vi "move.vi"(8 "error in (no error)":errorcluster, 11 "StageMG100204SutterMP285 in":refnum<class "StageMG100204SutterMP285.lvclass">=refnum) -> (0 "error out":errorcluster, 3 "StageMG100204SutterMP285 out":refnum<class "StageMG100204SutterMP285.lvclass">)   [LabVIEW 2010, in "StageMG100204SutterMP285.lvclass"]
uses:
  StageMG100204SutterMP285.lvclass
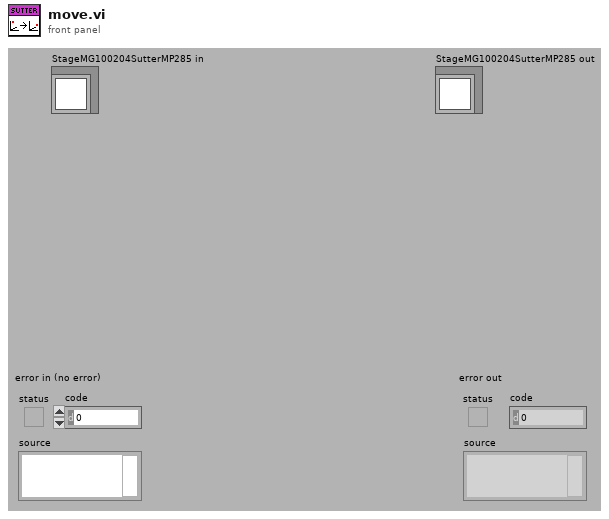
[diagram p1: front panel]
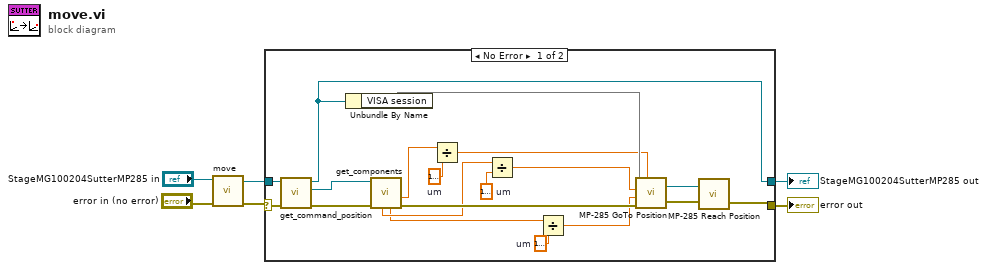
[diagram p0: block diagram]
diagram:
  n1 = call-parent "move.vi"("error in (no error)"="error in (no error)", "DL090409StageScaffold in"="StageMG100204SutterMP285 in") -> ("error out"=w5:errorcluster, "DL090409StageScaffold out"=w4:refnum<class "StageMG100204SutterMP285.lvclass">)  [unwired: 8 out]
  n2 = case shown="No Error" w5 {
    selector: w5 -> [w25 w27]
    tunnel: [w8 w27] -> w6
    tunnel: [w21 w26] -> w1
    tunnel: w4 -> [w24 w26]
    frame No Error {
      w15 = dbl[unit] 1e-06  # um
      w14 = dbl[unit] 1e-06  # um
      w18 = dbl[unit] 1e-06  # um
      n3 = call-dynamic "get_command_position.vi"("error in (no error)"=w25, "DL090409StageScaffold.lvclass in"=w24) -> ("error out"=w23:errorcluster, "SpaceVector.lvclass"=w22:refnum<class "SpaceVector.lvclass">, "DL090409StageScaffold.lvclass out"=w21:refnum<class "StageMG100204SutterMP285.lvclass">)  [unwired: 7 out]
      n4 = Unbundle By Name(w21) -> ("VISA session"=w20)
      n5 = call "get_components.vi"("error in (no error)"=w23, "SpaceVector in"=w22) -> ("error out"=w19:errorcluster, "x"=w17:dbl[unit], "z"=w11:dbl[unit], "y"=w13:dbl[unit])  [unwired: 6 out]
      n6 = Divide(x=w17, y=w18) -> (x/y=w16:dbl)
      n7 = Divide(x=w13, y=w14) -> (x/y=w12:dbl)
      n8 = Divide(x=w11, y=w15) -> (x/y=w10:dbl)
      n9 = call "MP-285 GoTo Position.vi"("VISA resource name"=w20, "Input: Y axis (microns)"=w12, "Input: Z axis (microns)"=w10, "error in (no error)"=w19, "Input: X axis (microns)"=w16) -> ("VISA resource name out"=w7:refnum<visa-resource-name>, "error out"=w9:errorcluster)
      n10 = call "MP-285 Reach Position.vi"("cluster"=w9, "Output: VISA session OUT"=w7) -> ("cluster 2"=w8:errorcluster)  [unwired: 1 out]
    }
    frame Error {
    }
  }
  "error out" <- w6
  "StageMG100204SutterMP285 out" <- w1
